vi "oa_Generate Waveform Reference with Vector Reference (N Channels).vi"(0 "resampled signal":cluster{"r0":dbl, "dr":dbl, "Y":dbl[]}[](array[cluster]) {"r0" format="%.2p"; "dr" format="%.2p"; "Y" format="%.2f"}, 1 "reset? (True)":bool=TRUE, 5 "slow roll vectors":cdb[][](array[numeric]) format="%.2f", 7 "orders to compensate":dbl[](array[numeric])=[1.0] format="%.2f", 9 "interpolated positions [s]":dbl[](array[numeric]), 11 "error out in":errorcluster) -> (4 "resampled signal out":cluster{"r0":dbl, "dr":dbl, "Y":dbl[]}[](array[cluster]) {"r0" format="%.2p"; "dr" format="%.2p"; "Y" format="%.2f"}, 6 "reference signal out":cluster{"r0":dbl, "dr":dbl, "Y":dbl[]}[](array[cluster]) {"r0" format="%.2p"; "dr" format="%.2p"; "Y" format="%.2f"}, 8 "slow roll vectors out":cdb[][](array[numeric]) format="%.2f", 15 "error out":errorcluster)   [LabVIEW 2017, in "SoundVib_RefDataProcess.lvlib"]
uses:
  <vilib>/addons/Sound and Vibration/Order Analysis/Referece Data Processing/SoundVib_RefDataProcess.lvlib
  <vilib>/Analysis/NI_AALBase.lvlib
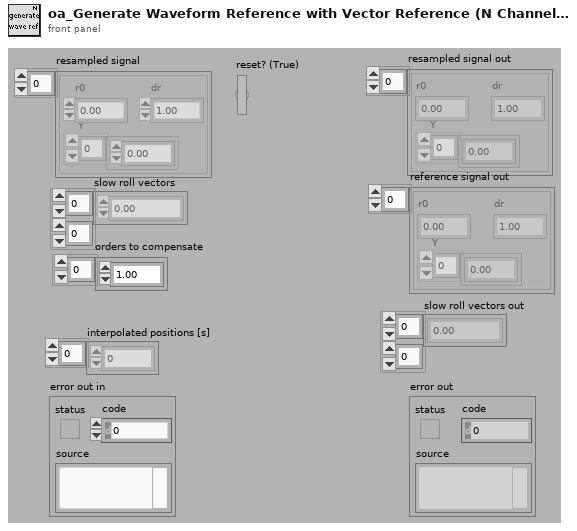
[diagram p1: front panel]
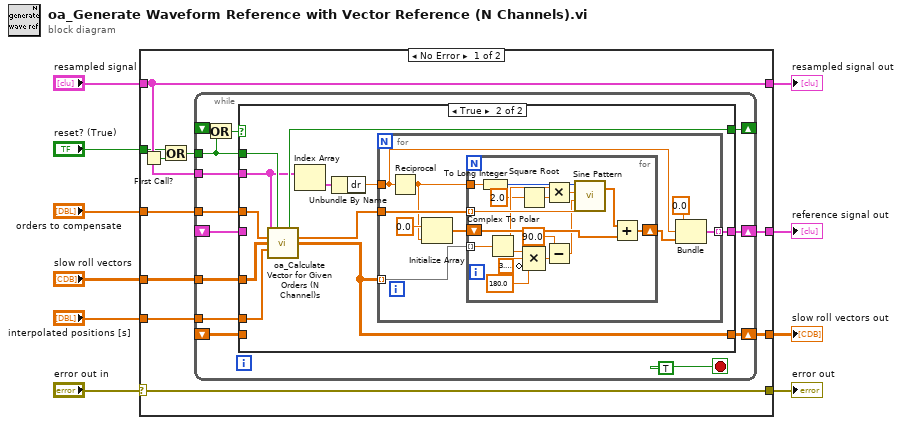
[diagram p0: block diagram]
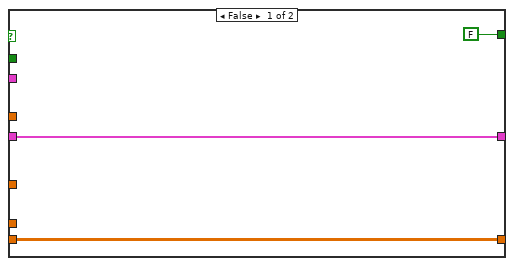
[diagram p2: hidden frame]
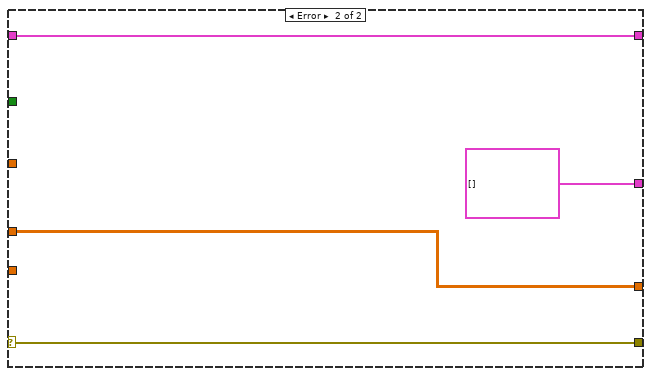
[diagram p3: hidden frame]
diagram:
  n1 = case shown="No Error" "error out in" {
    selector: "error out in" -> [w18 w77]
    tunnel: [w18 w77] -> w9
    tunnel: "reset? (True)" -> [w12 _]
    tunnel: "resampled signal" -> [w14 w76]
    tunnel: [w14 w76] -> w6
    tunnel: "orders to compensate" -> [w20 _]
    tunnel: "slow roll vectors" -> [w19 w74]
    tunnel: [w17 cluster{"r0":dbl, "dr":dbl, dbl[]}[] []] -> w3
    tunnel: "interpolated positions [s]" -> [w16 _]
    tunnel: [w11 w74] -> w1
    frame No Error {
      n2 = First Call?() -> (First Call?: T/F=w13:bool)
      n3 = Or(x=w12, y=w13) -> (x .or. y?=w15:bool)
      n4 = while {
        tunnel: w20 -> [w33]
        tunnel: w19 -> [w32]
        shift-right: [w30] -> w17
        shift-left: _ -> [w29]
        tunnel: w16 -> [w28]
        tunnel: w15 -> [w23]
        shift-right: [w27] -> _
        shift-left: _ -> [w25]
        tunnel: w14 -> [w26]
        shift-right: [w22] -> w11
        shift-left: _ -> [w21]
        stop <- TRUE stop-if-true
        n5 = Or(x=w25, y=w23) -> (x .or. y?=w24:bool)
        n6 = case shown="True" w24 {
          tunnel: w33 -> [_ w44]
          tunnel: w32 -> [_ w45]
          tunnel: [w36 w47] -> w30
          tunnel: w29 -> [w36 _]
          tunnel: w28 -> [_ w46]
          tunnel: w23 -> [_ w42]
          tunnel: [FALSE ("reset out") w41] -> w27
          tunnel: w26 -> [_ w39]
          tunnel: [w34 w37] -> w22
          tunnel: w21 -> [w34 _]
          frame False {
          }
          frame True {
            n7 = call <vilib>:"oa_Calculate Vector for Given Orders (N Channel)s.vi"("resampled signal"=w39, "reset? (True)"=w42, "orders to compensate"=w44, "slow roll vectors"=w45, "interpolated pulse positions"=w46) -> ("reset out"=w41:bool, "orders out"=w43:dbl[], "slow roll vectors"=w37:cdb[][])  [unwired: 7 in, 1 out]
            n8 = Index Array(array=w39) -> (element=w40:cluster{"r0":dbl, "dr":dbl, "Y":dbl[]})  [unwired: 1 in]
            n9 = Unbundle By Name(w40) -> ("dr"=w38:dbl)
            n10 = for {
              tunnel: w43 -> [w56]
              tunnel: w37 -> [w55] mode=indexing
              tunnel: w38 -> [w53]
              tunnel: [w54] -> w47 mode=indexing
              n11 = Reciprocal(x=w53) -> (1/x=w51:dbl)
              n12 = Initialize Array(0.0 ("element"), w51) -> (w50:dbl[])
              n13 = for {
                tunnel: w56 -> [w70] mode=indexing
                tunnel: w55 -> [w73] mode=indexing
                tunnel: w51 -> [w72]
                shift-right: [w68] -> w49
                shift-left: w50 -> [w67]
                n14 = To Long Integer(number=w72) -> (32bit integer=w71:i32)
                n15 = Complex To Polar(r * e^(i*theta)=w73) -> (r=w59:dbl, theta=w66:dbl)
                n16 = Square Root(x=2.0) -> (sqrt(x)=w58:dbl)
                n17 = Compound Arithmetic op=MULTIPLY(w66, 3.141592653589793, invert 180.0 ("value")) -> (w63:dbl)
                n18 = Multiply(x=w59, y=w58) -> (x*y=w60:dbl)
                n19 = Subtract(x=90.0, y=w63) -> (x-y=w61:dbl)
                n20 = call <vilib>:"Sine Pattern.vi"("cycles"=w70, "phase(degrees)"=w61, "amplitude"=w60, "samples"=w71) -> ("Sinusoidal Pattern"=w69:dbl[])  [unwired: 1 out]
                n21 = Add(x=w69, y=w67) -> (x+y=w68:dbl[])
              }
              n22 = Bundle("r0"=0.0, "dr"=w53, w49) -> (w54:cluster{"r0":dbl, "dr":dbl, dbl[]})  [unwired: 1 in]
            }
          }
        }
      }
    }
    frame Error {
    }
  }
  "error out" <- w9
  "resampled signal out" <- w6
  "reference signal out" <- w3
  "slow roll vectors out" <- w1
